vi "Main.vi"(8 "error in":errorcluster, 11 "TCP Listener in":refnum<class "TCP Listener.lvclass">) -> (0 "error out":errorcluster, 3 "TCP Listener out":refnum<class "TCP Listener.lvclass">)   [LabVIEW 2017, in "_TCP Server.lvlib" / "TCP Listener.lvclass"]
doc: "The <b>Queued Message Handler</b> of the Worker that owns this VI."
uses:
  TCP Listener.lvclass
  Initialization Data.ctl
  Response Cases.ctl
  <vilib>/addons/_Workers/Library/Case Label.ctl
  TCP Listener.lvclass/TCP Listener.ctl
  rqp_Listen for Connections.ctl
  rsp_Add Listener.ctl
  rsp_New Connection.ctl
  <vilib>/addons/_Workers/Library/Workers.lvlib
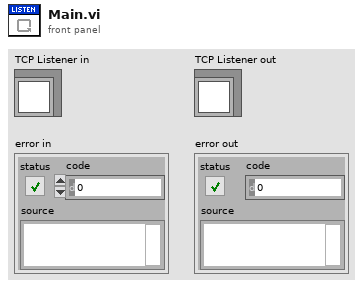
[diagram p1: front panel]
types:
  T1 = typedef "_TCP Server.lvlib/TCP Listener.lvclass/Initialization Data.ctl" = cluster{"Response Cases":T2}
  T2 = typedef "_TCP Server.lvlib/TCP Listener.lvclass/Response Cases.ctl" = cluster{"Add Listener":T3, "New Connection":T3}
  T3 = typedef "Workers.lvlib/Case Label.ctl" = string
  T4 = typedef "_TCP Server.lvlib/TCP Listener.lvclass/rsp_Add Listener.ctl" = cluster{"listener ID":refnum<k5>}
  T5 = typedef "_TCP Server.lvlib/TCP Listener.lvclass/rqp_Listen for Connections.ctl" = cluster{"Server Name":string, "Server IP Address":u32, "Server Port":u16}
  T6 = typedef "_TCP Server.lvlib/TCP Listener.lvclass/rsp_New Connection.ctl" = cluster{"Connection ID":refnum<k5>, "Client Name":string, "IP Address":string}
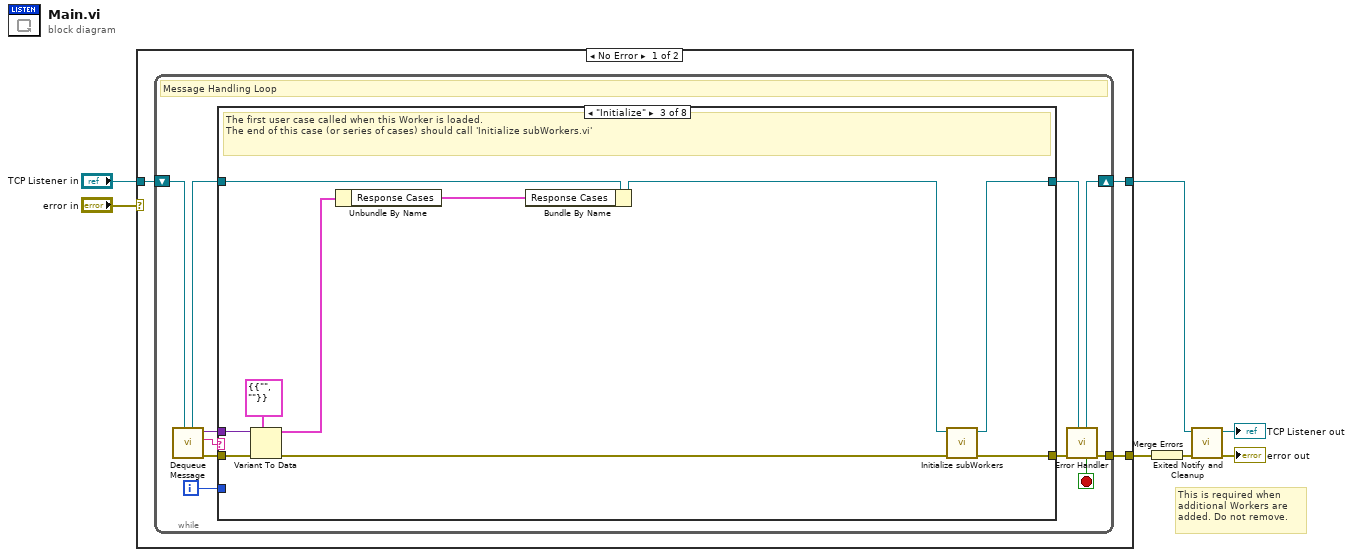
[diagram p0: block diagram]
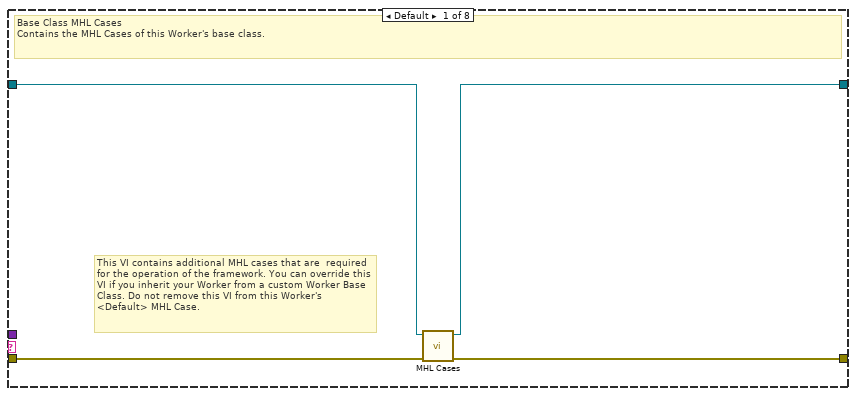
[diagram p2: hidden frame]
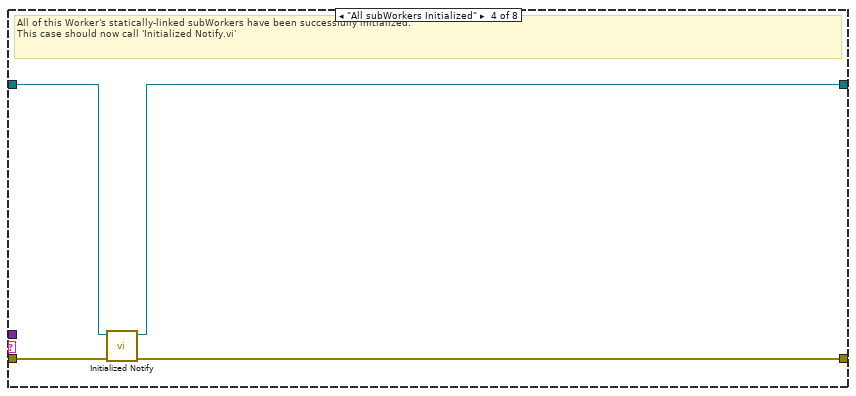
[diagram p4: hidden frame]
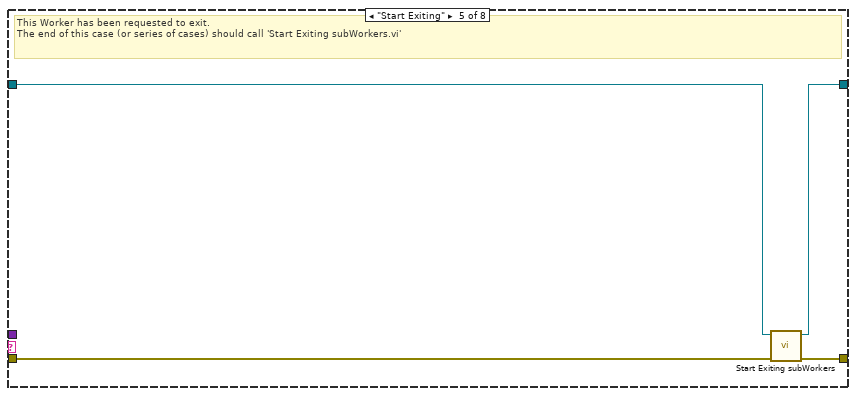
[diagram p5: hidden frame]
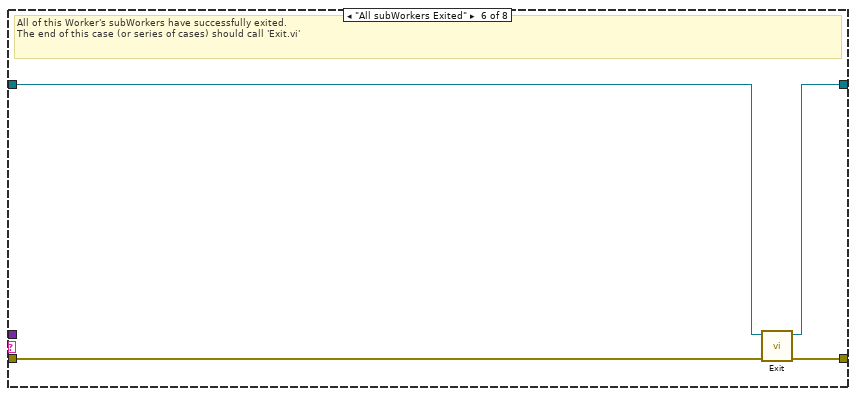
[diagram p6: hidden frame]
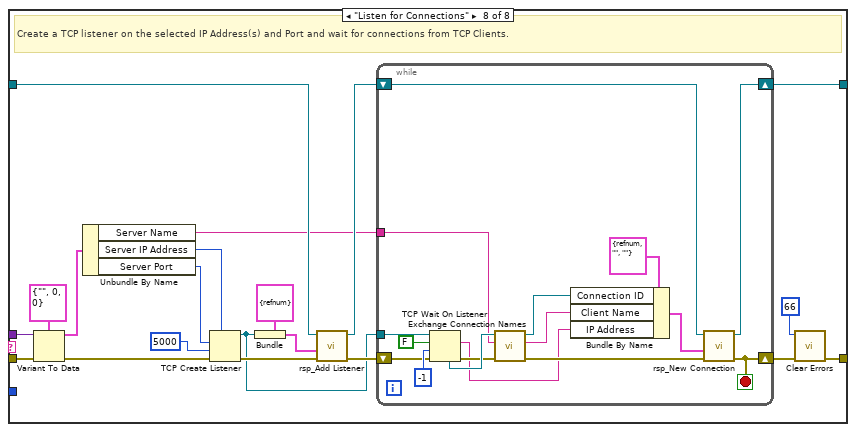
[diagram p8: hidden frame]
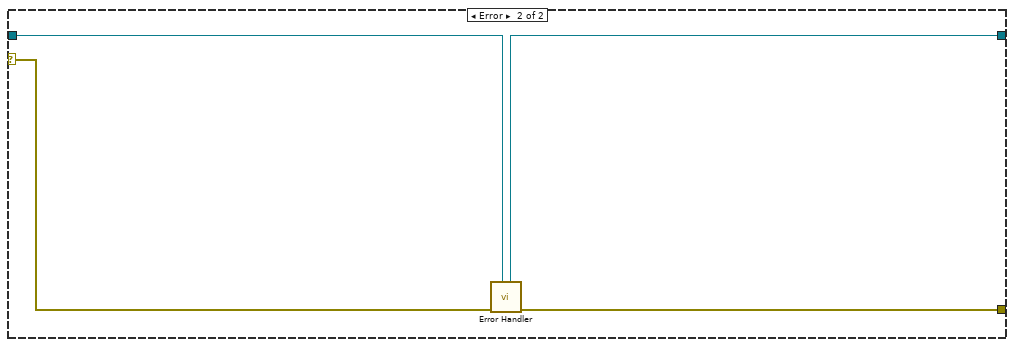
[diagram p9: hidden frame]
diagram:
  # "This is required when additional Workers are added. Do not remove."
  n1 = case shown="No Error" "error in" {
    tunnel: "TCP Listener in" -> [w8 w89]
    tunnel: [w10 w90] -> w6
    tunnel: [w9 w88] -> w7
    selector: "error in" -> [_ w91]
    frame No Error {
      n2 = while {
        shift-right: [w19] -> w9
        shift-left: w8 -> [w21]
        tunnel: [w20] -> w10
        i -> [w12]
        stop <- w13 stop-if-true
        # "Message Handling Loop"
        n3 = call-dynamic "Dequeue Message.vi"("Worker"=w21) -> ("error out"=w18:errorcluster, "Case out"=w14:string, "Data out"=w11:variant, "Worker out"=w16:refnum<class "TCP Listener.lvclass">)  [unwired: 6 in, 1 out]
        n4 = case "Worker MHL Case Structure (DO NOT CHANGE LABEL NAME)" shown="\"Initialize\"" w14 {
          tunnel: w18 -> [w25 w26 w35 w41 w42 w49 w51 w71]
          tunnel: [w24 w26 w37 w40 w45 w48 w51 w52] -> w17
          tunnel: w16 -> [w23 w27 w34 w39 w43 w47 w50 w67]
          tunnel: [w22 w27 w36 w38 w44 w46 w50 w59] -> w15
          tunnel: w12 -> [_ _ _ _ _ _ _ _]
          tunnel: w11 -> [_ _ w32 _ _ _ _ w69]
          frame Default {
            # "This VI contains additional MHL cases that are  required for the operation of the framework. You can override this VI if you inherit your Worker from a custom Worker Base Class. Do not remove this VI from this Worker's <Default> MHL Case."
            # "Base Class MHL Cases\nContains the MHL Cases of this Worker's base class."
            n5 = call-dynamic "MHL Cases.vi"("error in"=w25, "Worker in"=w23) -> ("error out"=w24:errorcluster, "Worker out"=w22:refnum<class "TCP Listener.lvclass">)  [unwired: 8 in]
          }
          frame "------------ FRAMEWORK CASES -----------" {
            # "Start of Workers Framework Cases"
          }
          frame "Initialize" {
            # "The first user case called when this Worker is loaded.\nThe end of this case (or series of cases) should call 'Initialize subWorkers.vi'"
            n6 = Variant To Data(error in=w35, type=T1 {"Response Cases"={"Add Listener"="", "New Connection"=""}} ("Cluster"), Variant=w32) -> (data=w30:T1, error out=w33:errorcluster)
            n7 = Unbundle By Name(w30) -> ("Response Cases"=w29:T2)
            n8 = Bundle By Name(cluster=w34, "Response Cases"=w29) -> (w31:refnum<class "TCP Listener.lvclass">)
            n9 = call-dynamic "Initialize subWorkers.vi"("error in"=w33, "Worker"=w31) -> ("error out"=w37:errorcluster, "dup Worker out"=w36:refnum<class "TCP Listener.lvclass">)  [unwired: 8 in]
          }
          frame "All subWorkers Initialized" {
            # "All of this Worker's statically-linked subWorkers have been successfully initialized.\nThis case should now call 'Initialized Notify.vi'"
            n10 = call-dynamic "Initialized Notify.vi"("error in"=w41, "Worker"=w39) -> ("error out"=w40:errorcluster, "dup Worker out"=w38:refnum<class "TCP Listener.lvclass">)  [unwired: 8 in]
          }
          frame "Start Exiting" {
            # "This Worker has been requested to exit. \nThe end of this case (or series of cases) should call 'Start Exiting subWorkers.vi'"
            n11 = call-dynamic "Start Exiting subWorkers.vi"("error_in"=w42, "Worker"=w43) -> ("error out"=w45:errorcluster, "dup Worker out"=w44:refnum<class "TCP Listener.lvclass">)  [unwired: 8 in]
          }
          frame "All subWorkers Exited" {
            # "All of this Worker's subWorkers have successfully exited. \nThe end of this case (or series of cases) should call 'Exit.vi'"
            n12 = call-dynamic "Exit.vi"("error_in"=w49, "Worker"=w47) -> ("error out"=w48:errorcluster, "dup Worker out"=w46:refnum<class "TCP Listener.lvclass">)  [unwired: 8 in]
          }
          frame "------------- PUBLIC API CASES -------------" {
            # "Start of Workers Public API Cases"
          }
          frame "Listen for Connections" {
            # "Create a TCP listener on the selected IP Address(s) and Port and wait for connections from TCP Clients."
            n13 = Variant To Data(error in=w71, type=T5 {"Server Name"="", "Server IP Address"=0, "Server Port"=0} ("Data"), Variant=w69) -> (data=w68:T5, error out=w63:errorcluster)
            n14 = Unbundle By Name(w68) -> ("Server Name"=w55:string, "Server IP Address"=w61:u32, "Server Port"=w60:u16)
            n15 = TCP Create Listener(7:w61, 8:w63, 9:5000 ("timeout ms (25000)"), 10:w60) -> (0:w62:errorcluster, 3:w56:refnum<k5>)  [unwired: 2 out]
            n16 = Bundle(cluster=T4 {"listener ID"=refnum} ("Data in"), "listener ID"=w56) -> (w65:T4)
            n17 = call "rsp_Add Listener.vi"("error in"=w62, "Data in"=w65, "TCP Listener in"=w67) -> ("error out"=w57:errorcluster, "dup TCP Listener out"=w58:refnum<class "TCP Listener.lvclass">)  [unwired: 7 in]
            n18 = while {
              shift-right: [w79] -> w59
              shift-left: w58 -> [w80]
              shift-right: [w73] -> w53
              shift-left: w57 -> [w85]
              tunnel: w56 -> [w84]
              tunnel: w55 -> [w81]
              stop <- w73 stop-if-true
              n19 = TCP Wait On Listener(8:w85, 9:-1 ("timeout ms (wait forever: -1)"), 10:FALSE ("resolve remote address (T)"), 11:w84) -> (0:w82:errorcluster, 2:w76:string, 4:w83:refnum<k5>)  [unwired: 2 out]
              n20 = call "Exchange Connection Names.vi"("error in (no error)"=w82, "Server Name in"=w81, "connection ID"=w83) -> ("error out"=w78:errorcluster, "Client Name out"=w75:string, "connection out"=w74:refnum<k5>)  [unwired: 6 in]
              n21 = Bundle By Name(cluster=T6 {"Connection ID"=refnum, "Client Name"="", "IP Address"=""} ("Data in"), "Connection ID"=w74, "Client Name"=w75, "IP Address"=w76) -> (w72:T6)
              n22 = call "rsp_New Connection.vi"("error in"=w78, "Data in"=w72, "TCP Listener in"=w80) -> ("error out"=w73:errorcluster, "dup TCP Listener out"=w79:refnum<class "TCP Listener.lvclass">)  [unwired: 7 in]
            }
            n23 = call <vilib>:"Clear Errors.vi"("error in (no error)"=w53, "specific error code to clear (0: all)"=66) -> ("error out"=w52:errorcluster)  [unwired: 4 in, 1 out]
          }
        }
        n24 = call-dynamic "Error Handler.vi"("Worker"=w15, "error_in"=w17) -> ("error out"=w20:errorcluster, "Stop Loop"=w13:bool, "Worker out"=w19:refnum<class "TCP Listener.lvclass">)  [unwired: 7 in]
      }
    }
    frame Error {
      n25 = call-dynamic "Error Handler.vi"("Worker"=w89, "error_in"=w91) -> ("error out"=w90:errorcluster, "Worker out"=w88:refnum<class "TCP Listener.lvclass">)  [unwired: 7 in, 1 out]
    }
  }
  n26 = Merge Errors(w6) -> (w3:errorcluster)
  n27 = call-dynamic "Exited Notify and Cleanup.vi"("error_in"=w3, "Worker"=w7) -> ("error out"=→"error out":errorcluster, "dup Worker out"=→"TCP Listener out":refnum<class "TCP Listener.lvclass">)  [unwired: 8 in]
